vi "Yellow to Red 3.vi"   [LabVIEW 2019]
uses:
  Global Var.vi
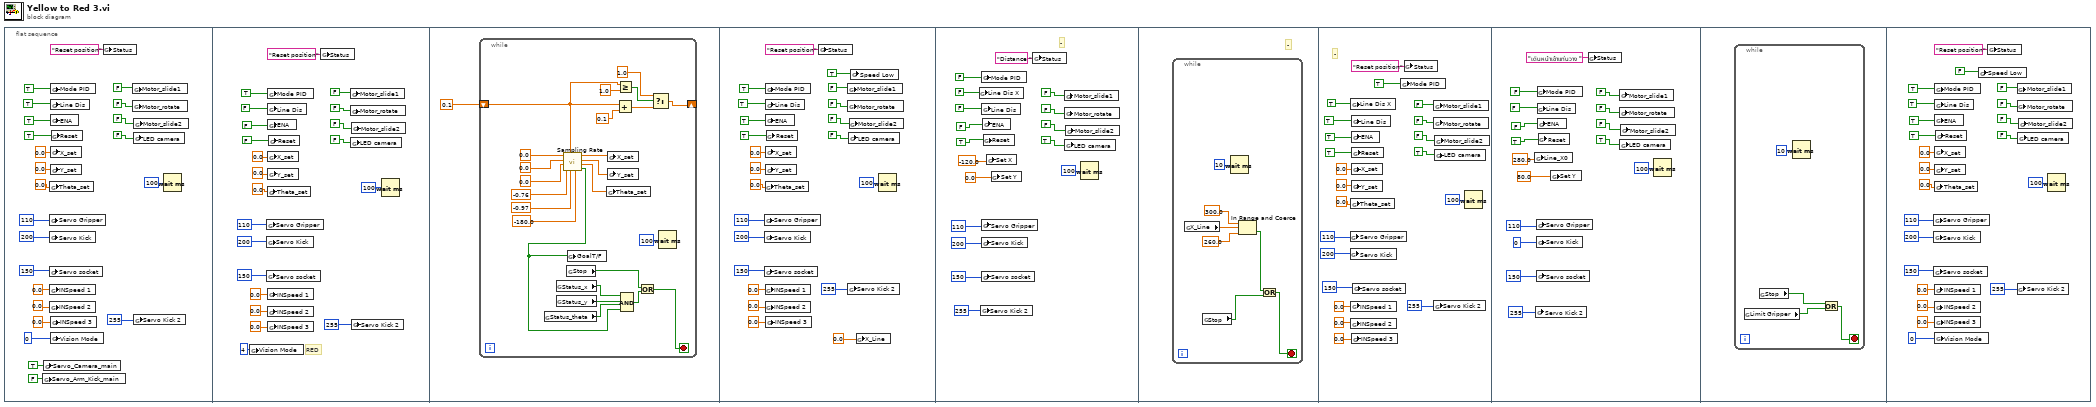
[diagram p0: block diagram]
diagram:
  n1 = flat-sequence {
    frame #0 {
      n2 = global write "Global Var.vi" "Servo_Arm_Kick_main"(FALSE ("Mode PID")) -> ()
      n3 = global write "Global Var.vi" "Servo_Camera_main"(TRUE ("Mode PID")) -> ()
      n4 = global write "Global Var.vi" "Servo Gripper"(u8 110 ("Servo Camera")) -> ()
      n5 = global write "Global Var.vi" "Servo Kick"(u8 200 ("Servo Camera")) -> ()
      n6 = global write "Global Var.vi" "Servo socket"(u8 150 ("Servo Camera")) -> ()
      n7 = global write "Global Var.vi" "Theta_set"(0.0 ("Theta_set")) -> ()
      n8 = global write "Global Var.vi" "INSpeed 1"(0.0 ("X_set")) -> ()
      n9 = global write "Global Var.vi" "INSpeed 2"(0.0 ("Y_set")) -> ()
      n10 = global write "Global Var.vi" "Mode PID"(TRUE ("Mode PID")) -> ()
      n11 = global write "Global Var.vi" "Line Dis"(TRUE ("Mode PID")) -> ()
      n12 = global write "Global Var.vi" "ENA"(TRUE ("ENA")) -> ()
      n13 = global write "Global Var.vi" "X_set"(0.0 ("X_set")) -> ()
      n14 = global write "Global Var.vi" "Y_set"(0.0 ("Y_set")) -> ()
      n15 = global write "Global Var.vi" "INSpeed 3"(0.0 ("Theta_set")) -> ()
      n16 = global write "Global Var.vi" "Vision Mode"(i16 0 ("Vision Mode")) -> ()
      n17 = global write "Global Var.vi" "Reset"(TRUE ("ENA")) -> ()
      n18 = global write "Global Var.vi" "Status"("Reset position" ("Status")) -> ()
      n19 = global write "Global Var.vi" "Motor_slide1"(FALSE ("Mode PID")) -> ()
      n20 = global write "Global Var.vi" "Motor_rotate"(FALSE ("ENA")) -> ()
      n21 = global write "Global Var.vi" "LED camera"(FALSE ("LED camera")) -> ()
      n22 = global write "Global Var.vi" "Motor_slide2"(FALSE ("ENA")) -> ()
      n23 = global write "Global Var.vi" "Servo Kick 2"(u8 255 ("Servo Camera")) -> ()
      n24 = Wait (ms)(milliseconds to wait=u32 100) -> ()  [unwired: 1 out]
    }
    frame #1 {
      # "RED"
      n25 = global write "Global Var.vi" "Vision Mode"(i16 4 ("Vision Mode")) -> ()
      n26 = global write "Global Var.vi" "Servo Gripper"(u8 110 ("Servo Camera")) -> ()
      n27 = global write "Global Var.vi" "Servo Kick"(u8 200 ("Servo Camera")) -> ()
      n28 = global write "Global Var.vi" "Servo socket"(u8 150 ("Servo Camera")) -> ()
      n29 = global write "Global Var.vi" "Theta_set"(0.0 ("Theta_set")) -> ()
      n30 = global write "Global Var.vi" "INSpeed 1"(0.0 ("X_set")) -> ()
      n31 = global write "Global Var.vi" "INSpeed 2"(0.0 ("Y_set")) -> ()
      n32 = global write "Global Var.vi" "Mode PID"(TRUE ("Mode PID")) -> ()
      n33 = global write "Global Var.vi" "Line Dis"(FALSE ("Mode PID")) -> ()
      n34 = global write "Global Var.vi" "ENA"(FALSE ("ENA")) -> ()
      n35 = global write "Global Var.vi" "X_set"(0.0 ("X_set")) -> ()
      n36 = global write "Global Var.vi" "Y_set"(0.0 ("Y_set")) -> ()
      n37 = global write "Global Var.vi" "INSpeed 3"(0.0 ("Theta_set")) -> ()
      n38 = global write "Global Var.vi" "Reset"(FALSE ("ENA")) -> ()
      n39 = global write "Global Var.vi" "Status"("Reset position" ("Status")) -> ()
      n40 = global write "Global Var.vi" "Motor_slide1"(FALSE ("Mode PID")) -> ()
      n41 = global write "Global Var.vi" "Motor_rotate"(FALSE ("ENA")) -> ()
      n42 = global write "Global Var.vi" "LED camera"(FALSE ("LED camera")) -> ()
      n43 = global write "Global Var.vi" "Motor_slide2"(FALSE ("ENA")) -> ()
      n44 = global write "Global Var.vi" "Servo Kick 2"(u8 255 ("Servo Camera")) -> ()
      n45 = Wait (ms)(milliseconds to wait=u32 100) -> ()  [unwired: 1 out]
    }
    frame #2 {
      n46 = while {
        shift-right: [w48] -> _
        shift-left: 0.1 -> [w46]
        stop <- w65 stop-if-true
        n47 = global read "Global Var.vi" "Status_theta"() -> (w67:bool)
        n48 = global read "Global Var.vi" "Status_x"() -> (w68:bool)
        n49 = global read "Global Var.vi" "Status_y"() -> (w69:bool)
        n50 = call "Sampling Rate.vi"("input a1"=-180.0, "input y1"=-0.97, "T(0-1)"=w46, "input x1"=-0.76, "input a0"=0.0, "input y0"=0.0, "input x0"=0.0) -> ("GoalT/F"=w53:bool, "a_output"=w60:dbl, "y_output"=w61:dbl, "x_output"=w62:dbl)  [unwired: 1 in]
        n51 = global read "Global Var.vi" "Stop"() -> (w63:bool)
        n52 = global write "Global Var.vi" "GoalT/F"(w53) -> ()
        n53 = global write "Global Var.vi" "Theta_set"(w60) -> ()
        n54 = global write "Global Var.vi" "X_set"(w62) -> ()
        n55 = global write "Global Var.vi" "Y_set"(w61) -> ()
        n56 = Add(x=w46, y=0.1) -> (x+y=w51:dbl)
        n57 = Greater Or Equal?(x=w46, y=1.0) -> (x >= y?=w50:bool)
        n58 = Compound Arithmetic op=AND(w68, w69, w67, w53) -> (w64:bool)
        n59 = Or(x=w63, y=w64) -> (x .or. y?=w65:bool)
        n60 = Select(t=1.0, s=w50, f=w51) -> (s? t:f=w48:dbl)
        n61 = Wait (ms)(milliseconds to wait=u32 100) -> ()  [unwired: 1 out]
      }
    }
    frame #3 {
      n62 = global write "Global Var.vi" "Servo Gripper"(u8 110 ("Servo Camera")) -> ()
      n63 = global write "Global Var.vi" "Servo Kick"(u8 200 ("Servo Camera")) -> ()
      n64 = global write "Global Var.vi" "Servo socket"(u8 150 ("Servo Camera")) -> ()
      n65 = global write "Global Var.vi" "Theta_set"(0.0 ("Theta_set")) -> ()
      n66 = global write "Global Var.vi" "INSpeed 1"(0.0 ("X_set")) -> ()
      n67 = global write "Global Var.vi" "INSpeed 2"(0.0 ("Y_set")) -> ()
      n68 = global write "Global Var.vi" "Mode PID"(TRUE ("Mode PID")) -> ()
      n69 = global write "Global Var.vi" "Line Dis"(TRUE ("Mode PID")) -> ()
      n70 = global write "Global Var.vi" "ENA"(TRUE ("ENA")) -> ()
      n71 = global write "Global Var.vi" "X_set"(0.0 ("X_set")) -> ()
      n72 = global write "Global Var.vi" "Y_set"(0.0 ("Y_set")) -> ()
      n73 = global write "Global Var.vi" "INSpeed 3"(0.0 ("Theta_set")) -> ()
      n74 = global write "Global Var.vi" "Reset"(TRUE ("ENA")) -> ()
      n75 = global write "Global Var.vi" "Status"("Reset position" ("Status")) -> ()
      n76 = global write "Global Var.vi" "Motor_slide1"(FALSE ("Mode PID")) -> ()
      n77 = global write "Global Var.vi" "Motor_rotate"(FALSE ("ENA")) -> ()
      n78 = global write "Global Var.vi" "Servo Kick 2"(u8 255 ("Servo Camera")) -> ()
      n79 = global write "Global Var.vi" "LED camera"(FALSE ("LED camera")) -> ()
      n80 = global write "Global Var.vi" "Motor_slide2"(FALSE ("ENA")) -> ()
      n81 = global write "Global Var.vi" "Speed Low"(TRUE ("Mode PID")) -> ()
      n82 = global write "Global Var.vi" "X_Line"(0.0 ("X_set")) -> ()
      n83 = Wait (ms)(milliseconds to wait=u32 100) -> ()  [unwired: 1 out]
    }
    frame #4 {
      # "-"
      n84 = global write "Global Var.vi" "Line Dis X"(FALSE ("Mode PID")) -> ()
      n85 = global write "Global Var.vi" "Servo Kick 2"(u8 255 ("Servo Camera")) -> ()
      n86 = global write "Global Var.vi" "Mode PID"(FALSE ("Mode PID")) -> ()
      n87 = global write "Global Var.vi" "Servo Gripper"(u8 110 ("Servo Camera")) -> ()
      n88 = global write "Global Var.vi" "Servo Kick"(u8 200 ("Servo Camera")) -> ()
      n89 = global write "Global Var.vi" "Servo socket"(u8 150 ("Servo Camera")) -> ()
      n90 = global write "Global Var.vi" "Line Dis"(FALSE ("Mode PID")) -> ()
      n91 = global write "Global Var.vi" "ENA"(FALSE ("ENA")) -> ()
      n92 = global write "Global Var.vi" "Reset"(TRUE ("ENA")) -> ()
      n93 = global write "Global Var.vi" "Set X"(-120.0 ("Y_set")) -> ()
      n94 = global write "Global Var.vi" "Set Y"(0.0 ("Y_set")) -> ()
      n95 = global write "Global Var.vi" "Status"("Distance " ("Status")) -> ()
      n96 = global write "Global Var.vi" "Motor_slide1"(FALSE ("Mode PID")) -> ()
      n97 = global write "Global Var.vi" "Motor_rotate"(FALSE ("ENA")) -> ()
      n98 = global write "Global Var.vi" "LED camera"(TRUE ("LED camera")) -> ()
      n99 = global write "Global Var.vi" "Motor_slide2"(FALSE ("ENA")) -> ()
      n100 = Wait (ms)(milliseconds to wait=u32 100) -> ()  [unwired: 1 out]
    }
    frame #5 {
      # "-"
      n101 = while {
        stop <- w114 stop-if-true
        n102 = global read "Global Var.vi" "X_Line"() -> (w112:dbl)
        n103 = global read "Global Var.vi" "Stop"() -> (w113:bool)
        n104 = Wait (ms)(milliseconds to wait=u32 10) -> ()  [unwired: 1 out]
        n105 = In Range and Coerce(upper limit=300.0, x=w112, lower limit=260.0) -> (In Range?=w109:bool)  [unwired: 1 out]
        n106 = Or(x=w109, y=w113) -> (x .or. y?=w114:bool)
      }
    }
    frame #6 {
      # "-"
      n107 = global write "Global Var.vi" "Servo Gripper"(u8 110 ("Servo Camera")) -> ()
      n108 = global write "Global Var.vi" "Servo Kick"(u8 200 ("Servo Camera")) -> ()
      n109 = global write "Global Var.vi" "Line Dis X"(TRUE ("Mode PID")) -> ()
      n110 = global write "Global Var.vi" "Theta_set"(0.0 ("Theta_set")) -> ()
      n111 = global write "Global Var.vi" "INSpeed 1"(0.0 ("X_set")) -> ()
      n112 = global write "Global Var.vi" "INSpeed 2"(0.0 ("Y_set")) -> ()
      n113 = global write "Global Var.vi" "Line Dis"(TRUE ("Mode PID")) -> ()
      n114 = global write "Global Var.vi" "ENA"(TRUE ("ENA")) -> ()
      n115 = global write "Global Var.vi" "X_set"(0.0 ("X_set")) -> ()
      n116 = global write "Global Var.vi" "Y_set"(0.0 ("Y_set")) -> ()
      n117 = global write "Global Var.vi" "INSpeed 3"(0.0 ("Theta_set")) -> ()
      n118 = global write "Global Var.vi" "Reset"(TRUE ("ENA")) -> ()
      n119 = global write "Global Var.vi" "Servo socket"(u8 150 ("Servo Camera")) -> ()
      n120 = global write "Global Var.vi" "Mode PID"(TRUE ("Mode PID")) -> ()
      n121 = global write "Global Var.vi" "Status"("Reset position" ("Status")) -> ()
      n122 = global write "Global Var.vi" "Motor_slide1"(FALSE ("Mode PID")) -> ()
      n123 = global write "Global Var.vi" "Motor_rotate"(FALSE ("ENA")) -> ()
      n124 = global write "Global Var.vi" "Servo Kick 2"(u8 255 ("Servo Camera")) -> ()
      n125 = global write "Global Var.vi" "LED camera"(TRUE ("LED camera")) -> ()
      n126 = global write "Global Var.vi" "Motor_slide2"(FALSE ("ENA")) -> ()
      n127 = Wait (ms)(milliseconds to wait=u32 100) -> ()  [unwired: 1 out]
    }
    frame #7 {
      n128 = global write "Global Var.vi" "Line_X0"(280.0 ("Y_set")) -> ()
      n129 = global write "Global Var.vi" "Servo Kick 2"(u8 255 ("Servo Camera")) -> ()
      n130 = global write "Global Var.vi" "Servo Gripper"(u8 110 ("Servo Camera")) -> ()
      n131 = global write "Global Var.vi" "Servo Kick"(u8 0 ("Servo Camera")) -> ()
      n132 = global write "Global Var.vi" "Servo socket"(u8 150 ("Servo Camera")) -> ()
      n133 = global write "Global Var.vi" "Mode PID"(FALSE ("Mode PID")) -> ()
      n134 = global write "Global Var.vi" "Line Dis"(FALSE ("Mode PID")) -> ()
      n135 = global write "Global Var.vi" "ENA"(FALSE ("ENA")) -> ()
      n136 = global write "Global Var.vi" "Reset"(TRUE ("ENA")) -> ()
      n137 = global write "Global Var.vi" "Set Y"(80.0 ("Y_set")) -> ()
      n138 = global write "Global Var.vi" "Status"("เดินหน้าเข้าแท่นวาง " ("Status")) -> ()
      n139 = global write "Global Var.vi" "Motor_slide1"(FALSE ("Mode PID")) -> ()
      n140 = global write "Global Var.vi" "Motor_rotate"(FALSE ("ENA")) -> ()
      n141 = global write "Global Var.vi" "LED camera"(TRUE ("LED camera")) -> ()
      n142 = global write "Global Var.vi" "Motor_slide2"(FALSE ("ENA")) -> ()
      n143 = Wait (ms)(milliseconds to wait=u32 100) -> ()  [unwired: 1 out]
    }
    frame #8 {
      n144 = while {
        stop <- w155 stop-if-true
        n145 = global read "Global Var.vi" "Limit Gripper"() -> (w153:bool)
        n146 = global read "Global Var.vi" "Stop"() -> (w154:bool)
        n147 = Wait (ms)(milliseconds to wait=u32 10) -> ()  [unwired: 1 out]
        n148 = Or(x=w154, y=w153) -> (x .or. y?=w155:bool)
      }
    }
    frame #9 {
      n149 = global write "Global Var.vi" "Servo Gripper"(u8 110 ("Servo Camera")) -> ()
      n150 = global write "Global Var.vi" "Servo Kick"(u8 200 ("Servo Camera")) -> ()
      n151 = global write "Global Var.vi" "Servo socket"(u8 150 ("Servo Camera")) -> ()
      n152 = global write "Global Var.vi" "Theta_set"(0.0 ("Theta_set")) -> ()
      n153 = global write "Global Var.vi" "INSpeed 1"(0.0 ("X_set")) -> ()
      n154 = global write "Global Var.vi" "INSpeed 2"(0.0 ("Y_set")) -> ()
      n155 = global write "Global Var.vi" "Mode PID"(TRUE ("Mode PID")) -> ()
      n156 = global write "Global Var.vi" "Line Dis"(TRUE ("Mode PID")) -> ()
      n157 = global write "Global Var.vi" "ENA"(TRUE ("ENA")) -> ()
      n158 = global write "Global Var.vi" "X_set"(0.0 ("X_set")) -> ()
      n159 = global write "Global Var.vi" "Y_set"(0.0 ("Y_set")) -> ()
      n160 = global write "Global Var.vi" "INSpeed 3"(0.0 ("Theta_set")) -> ()
      n161 = global write "Global Var.vi" "Vision Mode"(i16 0 ("Vision Mode")) -> ()
      n162 = global write "Global Var.vi" "Reset"(TRUE ("ENA")) -> ()
      n163 = global write "Global Var.vi" "Speed Low"(FALSE ("Mode PID")) -> ()
      n164 = global write "Global Var.vi" "Status"("Reset position" ("Status")) -> ()
      n165 = global write "Global Var.vi" "Motor_slide1"(FALSE ("Mode PID")) -> ()
      n166 = global write "Global Var.vi" "Motor_rotate"(FALSE ("ENA")) -> ()
      n167 = global write "Global Var.vi" "Servo Kick 2"(u8 255 ("Servo Camera")) -> ()
      n168 = global write "Global Var.vi" "LED camera"(FALSE ("LED camera")) -> ()
      n169 = global write "Global Var.vi" "Motor_slide2"(FALSE ("ENA")) -> ()
      n170 = Wait (ms)(milliseconds to wait=u32 100) -> ()  [unwired: 1 out]
    }
  }
